vi "LEDC Control Loop 2936 Main.vi"(0 "LEDAD Port":refnum<visa-resource-name>="COM7", 1 "Enable":u8, 2 "Inten Desired":refnum<vi>, 3 "Illum Meas":refnum<vi>, 5 "Light Meter Port":refnum<visa-resource-name>="COM4", 7 "Illum Desired":dbl, 9 "Error Margin":dbl=2.0, 11 "error in (no error)":errorcluster, 12 "Illum Cal Factor":dbl=3.62982 format="%#.6f", 13 "Channel":enum16{"Chn1", "Chn2"}(ring)) -> (4 "LEDAD Port out":refnum<visa-resource-name>, 6 "Light Meter Port out":refnum<visa-resource-name>, 8 "Illum Meas":dbl format="%#_4g", 10 "Inten Desired":dbl, 14 "Done":bool, 15 "error out":errorcluster)   [LabVIEW 2010]
panel:
  out "Flag2":bool
  out "Flag1":bool
  out "Slope":dbl format="%#_4g"
  in  "Illum 10":dbl format="%#_4g"
  in  "Stop":bool
  out "In Progress":bool
  in  "Illum 90":dbl format="%#_4g"
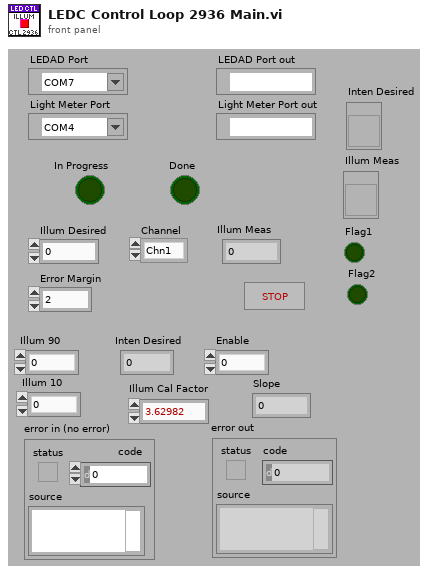
[diagram p1: front panel]
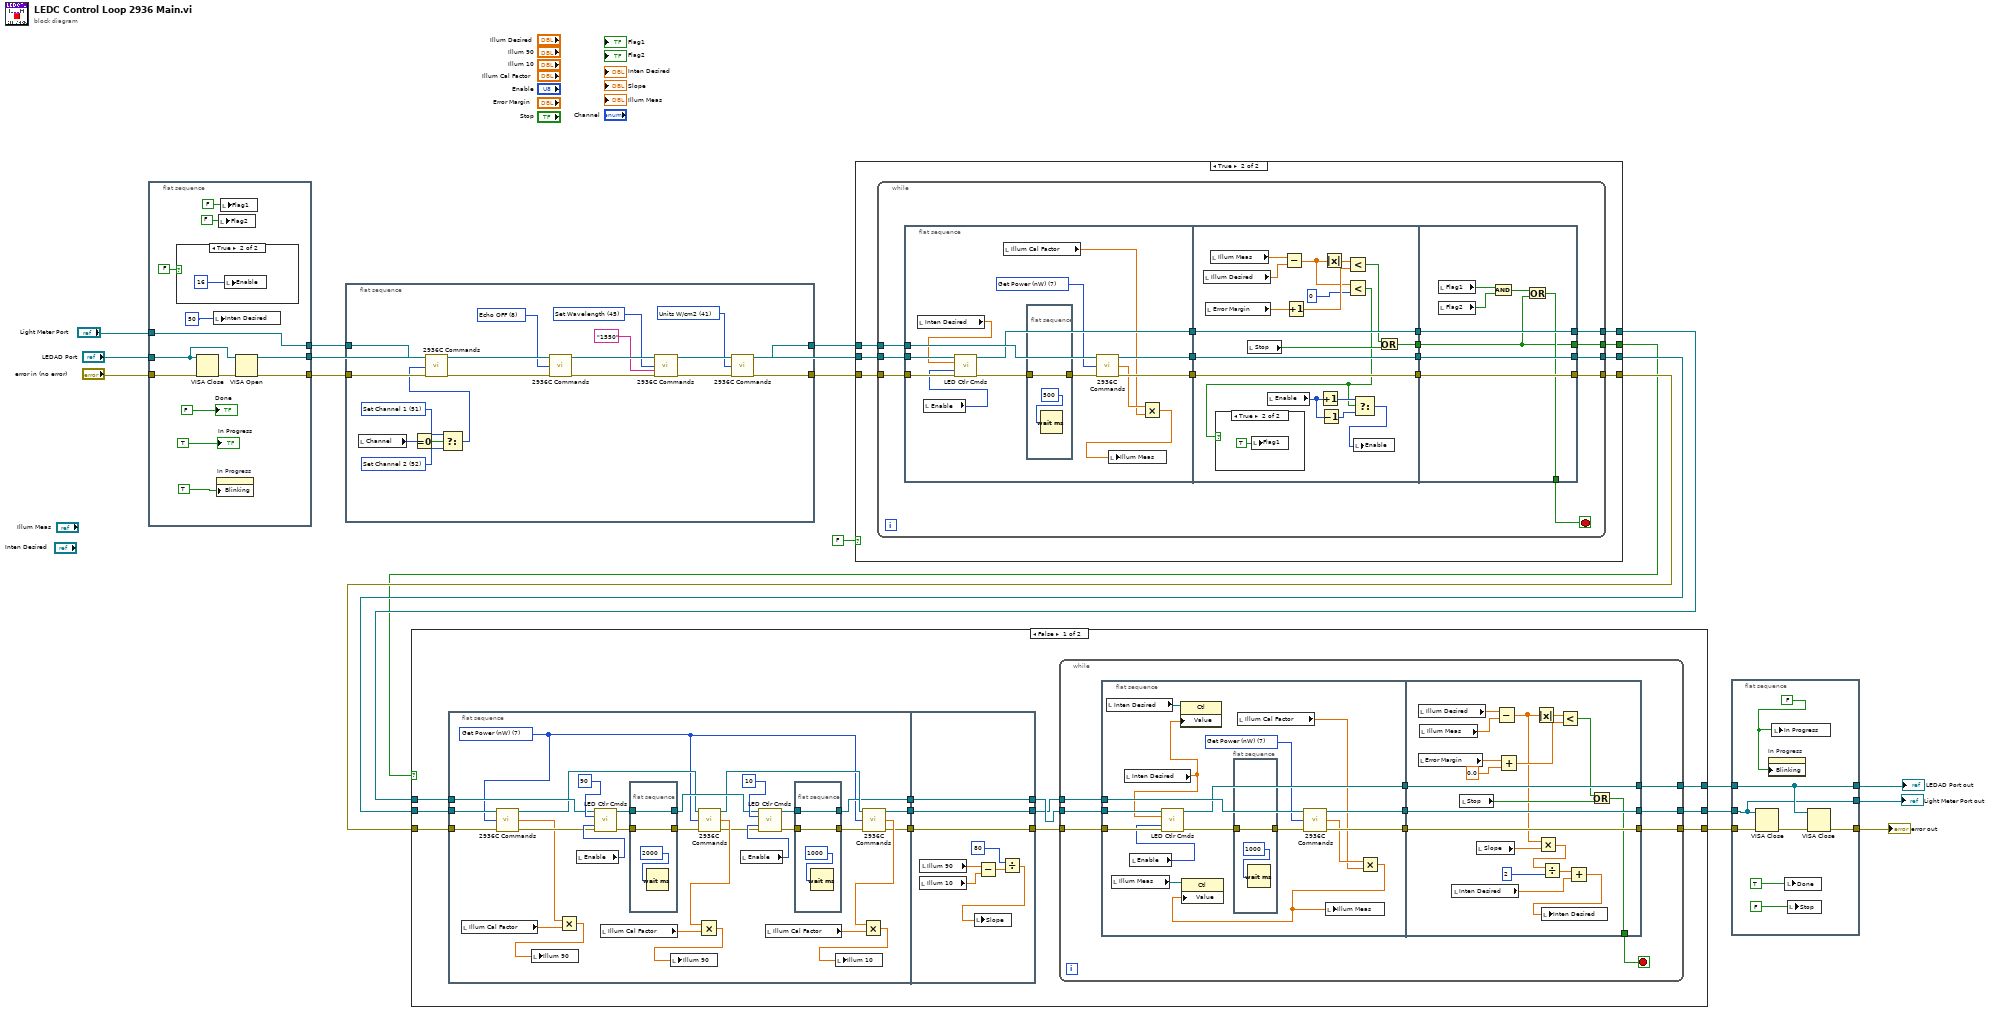
[diagram p0: block diagram]
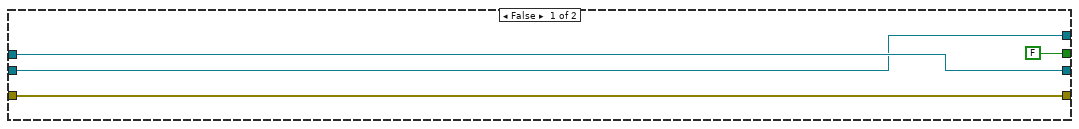
[diagram p2: hidden frame]
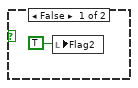
[diagram p3: hidden frame]
diagram:
  n1 = flat-sequence {
    tunnel: "LEDAD Port" -> [w25]
    tunnel: [w27] -> w3
    tunnel: "error in (no error)" -> [w28]
    tunnel: [w26] -> w18
    tunnel: "Light Meter Port" -> [w24]
    tunnel: [w24] -> w4
    frame #0 {
      n2 = case shown="True" FALSE {
        frame False {
        }
        frame True {
          n3 = local write "Enable"(16) -> ()
        }
      }
      n4 = VISA Close(VISA resource name=w25, error in (no error)=w28) -> (error out=w29:errorcluster)
      n5 = local write "Inten Desired"(50) -> ()
      n6 = property on="In Progress" class="Bool (strict)"("Blinking"=TRUE) -> ()  [unwired: 2 in, 2 out]
      n7 = local write "Flag2"(FALSE) -> ()
      n8 = local write "Flag1"(FALSE) -> ()
      n9 = VISA Open(error in (no error)=w29, VISA resource name=w25) -> (VISA resource name=w26:refnum<visa-resource-name>, error out=w27:errorcluster)  [unwired: 3 in]
      "Done" <- FALSE
      "In Progress" <- TRUE
    }
  }
  n10 = flat-sequence {
    tunnel: w3 -> [w52]
    tunnel: [w34] -> w1
    tunnel: w4 -> [w46]
    tunnel: [w35] -> w2
    frame #0 {
      w38 = u16 8 items=["Attenuator OFF", "Attenuator ON", "Attenuator Query", "Beep OFF", "Beep ON", "Beep Query", "Clear Status Reg", "Get Power (nW)", "Echo OFF", "Echo ON", "Echo Query", "No Filter", "Analog Filter", "Digital FIlter", "Filter Query", "Hold", "Go", "Go Query", "Backlight OFF", "Backlight Medium", "Backlight High", "Backlight Query", "Set Dsplay Screen 0", "Set Display Screen 1", "Display Screen Query", "Mode DC Continuous", "Mode DC Single", "Mode Integrate", "Identification", "Auto Range", "Auto Range Query", "Signal Range 0", "Signal Range 1", "Signal Range 2", "Signal Range 3", "Signal Range 4", "Signal Range 5", "Signal Range 6", "Signal Range Query", "Store Reference", "Units W", "Units W/cm2", "Units dBm", "Units Joules", "Units Query", "Set Wavelength", "Wavelength Querry", "Mode Pesk-to-Peak Cont.", "Mode Peak-to-Peak Sing.", "Mode Query", "Channel Querry", "Set Channel 1", "Set Channel 2"] ("Command")
      w41 = u16 41 items=["Attenuator OFF", "Attenuator ON", "Attenuator Query", "Beep OFF", "Beep ON", "Beep Query", "Clear Status Reg", "Get Power (nW)", "Echo OFF", "Echo ON", "Echo Query", "No Filter", "Analog Filter", "Digital FIlter", "Filter Query", "Hold", "Go", "Go Query", "Backlight OFF", "Backlight Medium", "Backlight High", "Backlight Query", "Set Dsplay Screen 0", "Set Display Screen 1", "Display Screen Query", "Mode DC Continuous", "Mode DC Single", "Mode Integrate", "Identification", "Auto Range", "Auto Range Query", "Signal Range 0", "Signal Range 1", "Signal Range 2", "Signal Range 3", "Signal Range 4", "Signal Range 5", "Signal Range 6", "Signal Range Query", "Store Reference", "Units W", "Units W/cm2", "Units dBm", "Units Joules", "Units Query", "Set Wavelength", "Wavelength Querry", "Mode Pesk-to-Peak Cont.", "Mode Peak-to-Peak Sing.", "Mode Query", "Channel Querry", "Set Channel 1", "Set Channel 2"] ("Command")
      w43 = u16 45 items=["Attenuator OFF", "Attenuator ON", "Attenuator Query", "Beep OFF", "Beep ON", "Beep Query", "Clear Status Reg", "Get Power (nW)", "Echo OFF", "Echo ON", "Echo Query", "No Filter", "Analog Filter", "Digital FIlter", "Filter Query", "Hold", "Go", "Go Query", "Backlight OFF", "Backlight Medium", "Backlight High", "Backlight Query", "Set Dsplay Screen 0", "Set Display Screen 1", "Display Screen Query", "Mode DC Continuous", "Mode DC Single", "Mode Integrate", "Identification", "Auto Range", "Auto Range Query", "Signal Range 0", "Signal Range 1", "Signal Range 2", "Signal Range 3", "Signal Range 4", "Signal Range 5", "Signal Range 6", "Signal Range Query", "Store Reference", "Units W", "Units W/cm2", "Units dBm", "Units Joules", "Units Query", "Set Wavelength", "Wavelength Querry", "Mode Pesk-to-Peak Cont.", "Mode Peak-to-Peak Sing.", "Mode Query", "Channel Querry", "Set Channel 1", "Set Channel 2"] ("Command")
      w51 = u16 52 items=["Attenuator OFF", "Attenuator ON", "Attenuator Query", "Beep OFF", "Beep ON", "Beep Query", "Clear Status Reg", "Get Power (nW)", "Echo OFF", "Echo ON", "Echo Query", "No Filter", "Analog Filter", "Digital FIlter", "Filter Query", "Hold", "Go", "Go Query", "Backlight OFF", "Backlight Medium", "Backlight High", "Backlight Query", "Set Dsplay Screen 0", "Set Display Screen 1", "Display Screen Query", "Mode DC Continuous", "Mode DC Single", "Mode Integrate", "Identification", "Auto Range", "Auto Range Query", "Signal Range 0", "Signal Range 1", "Signal Range 2", "Signal Range 3", "Signal Range 4", "Signal Range 5", "Signal Range 6", "Signal Range Query", "Store Reference", "Units W", "Units W/cm2", "Units dBm", "Units Joules", "Units Query", "Set Wavelength", "Wavelength Querry", "Mode Pesk-to-Peak Cont.", "Mode Peak-to-Peak Sing.", "Mode Query", "Channel Querry", "Set Channel 1", "Set Channel 2"] ("Command")
      w50 = u16 51 items=["Attenuator OFF", "Attenuator ON", "Attenuator Query", "Beep OFF", "Beep ON", "Beep Query", "Clear Status Reg", "Get Power (nW)", "Echo OFF", "Echo ON", "Echo Query", "No Filter", "Analog Filter", "Digital FIlter", "Filter Query", "Hold", "Go", "Go Query", "Backlight OFF", "Backlight Medium", "Backlight High", "Backlight Query", "Set Dsplay Screen 0", "Set Display Screen 1", "Display Screen Query", "Mode DC Continuous", "Mode DC Single", "Mode Integrate", "Identification", "Auto Range", "Auto Range Query", "Signal Range 0", "Signal Range 1", "Signal Range 2", "Signal Range 3", "Signal Range 4", "Signal Range 5", "Signal Range 6", "Signal Range Query", "Store Reference", "Units W", "Units W/cm2", "Units dBm", "Units Joules", "Units Query", "Set Wavelength", "Wavelength Querry", "Mode Pesk-to-Peak Cont.", "Mode Peak-to-Peak Sing.", "Mode Query", "Channel Querry", "Set Channel 1", "Set Channel 2"] ("Command")
      n11 = local read "Channel"() -> (w48:enum16{"Chn1", "Chn2"})
      n12 = Equal To 0?(x=w48) -> (x = 0?=w49:bool)
      n13 = Select(t=w50, s=w49, f=w51) -> (s? t:f=w47:u16)
      n14 = call "2936C Commands.vi"("Instrument Resource Name"=w46, "Command"=w47, "error in (no error)"=w52) -> ("VISA resource name out"=w36:refnum<visa-resource-name>, "error out"=w37:errorcluster)  [unwired: 8 in, 3 out]
      n15 = call "2936C Commands.vi"("Instrument Resource Name"=w36, "Command"=w38, "error in (no error)"=w37) -> ("VISA resource name out"=w39:refnum<visa-resource-name>, "error out"=w40:errorcluster)  [unwired: 8 in, 3 out]
      n16 = call "2936C Commands.vi"("Instrument Resource Name"=w39, "Command"=w43, "Wavelength"="1550", "error in (no error)"=w40) -> ("VISA resource name out"=w45:refnum<visa-resource-name>, "error out"=w44:errorcluster)  [unwired: 7 in, 3 out]
      n17 = call "2936C Commands.vi"("Instrument Resource Name"=w45, "Command"=w41, "error in (no error)"=w44) -> ("VISA resource name out"=w35:refnum<visa-resource-name>, "error out"=w34:errorcluster)  [unwired: 8 in, 3 out]
    }
  }
  n18 = case shown="True" FALSE {
    tunnel: w18 -> [w55 w63]
    tunnel: w2 -> [w56 w62]
    tunnel: w1 -> [w54 w61]
    tunnel: [w55 w60] -> w14
    tunnel: [w56 w59] -> w13
    tunnel: [w54 w58] -> w12
    tunnel: [FALSE w57] -> w11
    frame False {
    }
    frame True {
      n19 = while {
        tunnel: w62 -> [w78]
        tunnel: w63 -> [w77]
        tunnel: w61 -> [w76]
        tunnel: [w69] -> w59
        tunnel: [w67] -> w58
        tunnel: [w68] -> w60
        tunnel: [w64] -> w57
        stop <- w65 stop-if-true
        n20 = flat-sequence {
          tunnel: w76 -> [w91]
          tunnel: w77 -> [w92]
          tunnel: w78 -> [w90]
          tunnel: [w89] -> w72
          tunnel: [w87] -> w71
          tunnel: [w88] -> w70
          tunnel: [w111] -> w75
          tunnel: [w110] -> w74
          tunnel: [w109] -> w73
          tunnel: w72 -> [w111]
          tunnel: w71 -> [w110]
          tunnel: w70 -> [w109]
          tunnel: [w96] -> w66
          tunnel: w75 -> [w122]
          tunnel: w74 -> [w121]
          tunnel: w73 -> [w120]
          tunnel: [w122] -> w69
          tunnel: [w121] -> w68
          tunnel: [w120] -> w67
          tunnel: w66 -> [w115]
          tunnel: [w116] -> w65
          tunnel: [w115] -> w64
          frame #0 {
            w79 = u16 7 items=["Attenuator OFF", "Attenuator ON", "Attenuator Query", "Beep OFF", "Beep ON", "Beep Query", "Clear Status Reg", "Get Power (nW)", "Echo OFF", "Echo ON", "Echo Query", "No Filter", "Analog Filter", "Digital FIlter", "Filter Query", "Hold", "Go", "Go Query", "Backlight OFF", "Backlight Medium", "Backlight High", "Backlight Query", "Set Dsplay Screen 0", "Set Display Screen 1", "Display Screen Query", "Mode DC Continuous", "Mode DC Single", "Mode Integrate", "Identification", "Auto Range", "Auto Range Query", "Signal Range 0", "Signal Range 1", "Signal Range 2", "Signal Range 3", "Signal Range 4", "Signal Range 5", "Signal Range 6", "Signal Range Query", "Store Reference", "Units W", "Units W/cm2", "Units dBm", "Units Joules", "Units Query", "Set Wavelength", "Wavelength Querry", "Mode Pesk-to-Peak Cont.", "Mode Peak-to-Peak Sing.", "Mode Query", "Channel Querry", "Set Channel 1", "Set Channel 2"] ("Command")
            n21 = local read "Inten Desired"() -> (w84:dbl)
            n22 = local read "Enable"() -> (w83:u8)
            n23 = call "LED Ctlr Cmds.vi"("VISA session"=w92, "Intensity"=w84, "Enable"=w83, "error in (no error)"=w91) -> ("VISA session out"=w87:refnum<visa-resource-name>, "error out"=w86:errorcluster)  [unwired: 7 in, 3 out]
            n24 = local read "Illum Cal Factor"() -> (w80:dbl)
            n25 = flat-sequence {
              tunnel: w86 -> [w94]
              tunnel: [w94] -> w85
              frame #0 {
                n26 = Wait (ms)(milliseconds to wait=500) -> ()  [unwired: 1 out]
              }
            }
            n27 = call "2936C Commands.vi"("Instrument Resource Name"=w90, "Command"=w79, "error in (no error)"=w85) -> ("VISA resource name out"=w89:refnum<visa-resource-name>, "LM Response"=w81:dbl, "error out"=w88:errorcluster)  [unwired: 8 in, 2 out]
            n28 = Multiply(x=w81, y=w80) -> (x*y=w82:dbl)
            n29 = local write "Illum Meas"(w82) -> ()
          }
          frame #1 {
            n30 = local read "Illum Desired"() -> (w106:dbl)
            n31 = local read "Error Margin"() -> (w104:dbl)
            n32 = local read "Illum Meas"() -> (w107:dbl)
            n33 = local read "Stop"() -> (w103:bool)
            n34 = local read "Enable"() -> (w98:u8)
            n35 = Subtract(x=w107, y=w106) -> (x-y=w102:dbl)
            n36 = Increment(x=w104) -> (x+1=w105:dbl)
            n37 = Increment(x=w98) -> (x+1=w99:u8)
            n38 = Decrement(x=w98) -> (x-1=w100:u8)
            n39 = Absolute Value(x=w102) -> (abs(x)=w112:dbl)
            n40 = Less?(x=w112, y=w105) -> (x < y?=w108:bool)
            n41 = Less?(x=w102, y=0) -> (x < y?=w97:bool)
            n42 = case shown="True" w97 {
              frame False {
                n43 = local write "Flag2"(TRUE) -> ()
              }
              frame True {
                n44 = local write "Flag1"(TRUE) -> ()
              }
            }
            n45 = Select(t=w99, s=w97, f=w100) -> (s? t:f=w95:u8)
            n46 = local write "Enable"(w95) -> ()
            n47 = Or(x=w108, y=w103) -> (x .or. y?=w96:bool)
          }
          frame #2 {
            n48 = local read "Flag1"() -> (w119:bool)
            n49 = local read "Flag2"() -> (w118:bool)
            n50 = And(x=w119, y=w118) -> (x .and. y?=w117:bool)
            n51 = Or(x=w117, y=w115) -> (x .or. y?=w116:bool)
          }
        }
      }
    }
  }
  n52 = case shown="False" w11 {
    tunnel: w14 -> [w126 w227]
    tunnel: w13 -> [w132 w228]
    tunnel: w12 -> [w131 w229]
    tunnel: [w127 w229] -> w10
    tunnel: [w129 w228] -> w9
    tunnel: [w128 w227] -> w8
    frame False {
      n53 = flat-sequence {
        tunnel: w132 -> [w142]
        tunnel: w131 -> [w141]
        tunnel: [w148] -> w134
        tunnel: [w147] -> w133
        tunnel: w126 -> [w146]
        tunnel: [w143] -> w125
        tunnel: [w179] -> w123
        tunnel: w134 -> [w179]
        tunnel: [w178] -> w130
        tunnel: w133 -> [w178]
        tunnel: [w174] -> w124
        tunnel: w125 -> [w174]
        frame #0 {
          w135 = u16 7 items=["Attenuator OFF", "Attenuator ON", "Attenuator Query", "Beep OFF", "Beep ON", "Beep Query", "Clear Status Reg", "Get Power (nW)", "Echo OFF", "Echo ON", "Echo Query", "No Filter", "Analog Filter", "Digital FIlter", "Filter Query", "Hold", "Go", "Go Query", "Backlight OFF", "Backlight Medium", "Backlight High", "Backlight Query", "Set Dsplay Screen 0", "Set Display Screen 1", "Display Screen Query", "Mode DC Continuous", "Mode DC Single", "Mode Integrate", "Identification", "Auto Range", "Auto Range Query", "Signal Range 0", "Signal Range 1", "Signal Range 2", "Signal Range 3", "Signal Range 4", "Signal Range 5", "Signal Range 6", "Signal Range Query", "Store Reference", "Units W", "Units W/cm2", "Units dBm", "Units Joules", "Units Query", "Set Wavelength", "Wavelength Querry", "Mode Pesk-to-Peak Cont.", "Mode Peak-to-Peak Sing.", "Mode Query", "Channel Querry", "Set Channel 1", "Set Channel 2"] ("Command")
          n54 = local read "Illum Cal Factor"() -> (w138:dbl)
          n55 = call "2936C Commands.vi"("Instrument Resource Name"=w142, "Command"=w135, "error in (no error)"=w141) -> ("VISA resource name out"=w140:refnum<visa-resource-name>, "LM Response"=w136:dbl, "error out"=w139:errorcluster)  [unwired: 8 in, 2 out]
          n56 = Multiply(x=w136, y=w138) -> (x*y=w137:dbl)
          n57 = local write "Illum 90"(w137) -> ()
          n58 = local read "Enable"() -> (w165:u8)
          n59 = call "LED Ctlr Cmds.vi"("VISA session"=w146, "Intensity"=90, "Enable"=w165, "error in (no error)"=w139) -> ("VISA session out"=w162:refnum<visa-resource-name>, "error out"=w163:errorcluster)  [unwired: 7 in, 3 out]
          n60 = local read "Illum Cal Factor"() -> (w158:dbl)
          n61 = flat-sequence {
            tunnel: w163 -> [w171]
            tunnel: [w171] -> w161
            tunnel: [w169] -> w145
            tunnel: w162 -> [w169]
            frame #0 {
              n62 = Wait (ms)(milliseconds to wait=2000) -> ()  [unwired: 1 out]
            }
          }
          n63 = call "2936C Commands.vi"("Instrument Resource Name"=w140, "Command"=w135, "error in (no error)"=w161) -> ("VISA resource name out"=w144:refnum<visa-resource-name>, "LM Response"=w159:dbl, "error out"=w149:errorcluster)  [unwired: 8 in, 2 out]
          n64 = Multiply(x=w159, y=w158) -> (x*y=w160:dbl)
          n65 = local write "Illum 90"(w160) -> ()
          n66 = local read "Enable"() -> (w150:u8)
          n67 = call "LED Ctlr Cmds.vi"("VISA session"=w145, "Intensity"=10, "Enable"=w150, "error in (no error)"=w149) -> ("VISA session out"=w153:refnum<visa-resource-name>, "error out"=w152:errorcluster)  [unwired: 7 in, 3 out]
          n68 = local read "Illum Cal Factor"() -> (w157:dbl)
          n69 = flat-sequence {
            tunnel: w152 -> [w168]
            tunnel: [w168] -> w154
            tunnel: [w166] -> w143
            tunnel: w153 -> [w166]
            frame #0 {
              n70 = Wait (ms)(milliseconds to wait=1000) -> ()  [unwired: 1 out]
            }
          }
          n71 = call "2936C Commands.vi"("Instrument Resource Name"=w144, "Command"=w135, "error in (no error)"=w154) -> ("VISA resource name out"=w148:refnum<visa-resource-name>, "LM Response"=w156:dbl, "error out"=w147:errorcluster)  [unwired: 8 in, 2 out]
          n72 = Multiply(x=w156, y=w157) -> (x*y=w155:dbl)
          n73 = local write "Illum 10"(w155) -> ()
        }
        frame #1 {
          n74 = local read "Illum 10"() -> (w176:dbl)
          n75 = local read "Illum 90"() -> (w177:dbl)
          n76 = Subtract(x=w177, y=w176) -> (x-y=w173:dbl)
          n77 = Divide(x=80, y=w173) -> (x/y=w175:dbl)
          n78 = local write "Slope"(w175) -> ()
        }
      }
      n79 = while {
        tunnel: w123 -> [w189]
        tunnel: w124 -> [w188]
        tunnel: w130 -> [w187]
        tunnel: [w183] -> w129
        tunnel: [w181] -> w127
        tunnel: [w182] -> w128
        stop <- w180 stop-if-true
        n80 = flat-sequence {
          tunnel: w187 -> [w204]
          tunnel: w188 -> [w205]
          tunnel: w189 -> [w203]
          tunnel: [w202] -> w186
          tunnel: [w200] -> w185
          tunnel: [w201] -> w184
          tunnel: w186 -> [w225]
          tunnel: w185 -> [w224]
          tunnel: w184 -> [w223]
          tunnel: [w210] -> w180
          tunnel: [w225] -> w183
          tunnel: [w224] -> w182
          tunnel: [w223] -> w181
          frame #0 {
            w190 = u16 7 items=["Attenuator OFF", "Attenuator ON", "Attenuator Query", "Beep OFF", "Beep ON", "Beep Query", "Clear Status Reg", "Get Power (nW)", "Echo OFF", "Echo ON", "Echo Query", "No Filter", "Analog Filter", "Digital FIlter", "Filter Query", "Hold", "Go", "Go Query", "Backlight OFF", "Backlight Medium", "Backlight High", "Backlight Query", "Set Dsplay Screen 0", "Set Display Screen 1", "Display Screen Query", "Mode DC Continuous", "Mode DC Single", "Mode Integrate", "Identification", "Auto Range", "Auto Range Query", "Signal Range 0", "Signal Range 1", "Signal Range 2", "Signal Range 3", "Signal Range 4", "Signal Range 5", "Signal Range 6", "Signal Range Query", "Store Reference", "Units W", "Units W/cm2", "Units dBm", "Units Joules", "Units Query", "Set Wavelength", "Wavelength Querry", "Mode Pesk-to-Peak Cont.", "Mode Peak-to-Peak Sing.", "Mode Query", "Channel Querry", "Set Channel 1", "Set Channel 2"] ("Command")
            n81 = local read "Inten Desired"() -> (w194:refnum<vi>)
            n82 = local read "Illum Meas"() -> (w192:refnum<vi>)
            n83 = local read "Inten Desired"() -> (w193:dbl)
            n84 = local read "Enable"() -> (w197:u8)
            n85 = call "LED Ctlr Cmds.vi"("VISA session"=w205, "Intensity"=w193, "Enable"=w197, "error in (no error)"=w204) -> ("VISA session out"=w200:refnum<visa-resource-name>, "error out"=w199:errorcluster)  [unwired: 7 in, 3 out]
            n86 = property class="Ctl"(reference=w194, "Value"=w193) -> ()  [unwired: 1 in, 2 out]
            n87 = flat-sequence {
              tunnel: w199 -> [w207]
              tunnel: [w207] -> w198
              frame #0 {
                n88 = Wait (ms)(milliseconds to wait=1000) -> ()  [unwired: 1 out]
              }
            }
            n89 = local read "Illum Cal Factor"() -> (w195:dbl)
            n90 = call "2936C Commands.vi"("Instrument Resource Name"=w203, "Command"=w190, "error in (no error)"=w198) -> ("VISA resource name out"=w202:refnum<visa-resource-name>, "LM Response"=w196:dbl, "error out"=w201:errorcluster)  [unwired: 8 in, 2 out]
            n91 = Multiply(x=w196, y=w195) -> (x*y=w191:dbl)
            n92 = property class="Ctl"(reference=w192, "Value"=w191) -> ()  [unwired: 1 in, 2 out]
            n93 = local write "Illum Meas"(w191) -> ()
          }
          frame #1 {
            n94 = local read "Error Margin"() -> (w209:dbl)
            n95 = local read "Illum Desired"() -> (w221:dbl)
            n96 = local read "Illum Meas"() -> (w220:dbl)
            n97 = local read "Inten Desired"() -> (w212:dbl)
            n98 = local read "Stop"() -> (w218:bool)
            n99 = local read "Slope"() -> (w216:dbl)
            n100 = Subtract(x=w221, y=w220) -> (x-y=w214:dbl)
            n101 = Add(x=w209, y=0.0) -> (x+y=w219:dbl)
            n102 = Absolute Value(x=w214) -> (abs(x)=w226:dbl)
            n103 = Multiply(x=w214, y=w216) -> (x*y=w213:dbl)
            n104 = Divide(x=w213, y=2) -> (x/y=w215:dbl)
            n105 = Less?(x=w226, y=w219) -> (x < y?=w222:bool)
            n106 = Add(x=w215, y=w212) -> (x+y=w211:dbl)
            n107 = local write "Inten Desired"(w211) -> ()
            n108 = Or(x=w222, y=w218) -> (x .or. y?=w210:bool)
          }
        }
      }
    }
    frame True {
    }
  }
  n109 = flat-sequence {
    tunnel: w9 -> [w233]
    tunnel: w10 -> [w235]
    tunnel: [w234] -> w6
    tunnel: w8 -> [w234]
    tunnel: [w233] -> w7
    tunnel: [w231] -> w19
    frame #0 {
      w237 = FALSE
      n110 = VISA Close(VISA resource name=w233, error in (no error)=w235) -> (error out=w232:errorcluster)
      n111 = property on="In Progress" class="Bool (strict)"("Blinking"=w237) -> ()  [unwired: 2 in, 2 out]
      n112 = local write "In Progress"(w237) -> ()
      n113 = local write "Done"(TRUE) -> ()
      n114 = local write "Stop"(FALSE) -> ()
      n115 = VISA Close(VISA resource name=w234, error in (no error)=w232) -> (error out=w231:errorcluster)
    }
  }
  "error out" <- w19
  "Light Meter Port out" <- w7
  "LEDAD Port out" <- w6
